vi "toStringArray.vi"(8 "error in (no error)":errorcluster, 11 "ScriptEvent in":refnum<class "ScriptEvent.lvclass">) -> (0 "error out":errorcluster, 2 "eventStringArray":string[](array[string]), 3 "ScriptEvent out":refnum<class "ScriptEvent.lvclass">)   [LabVIEW 2011, in "Tools.lvlib" / "Scripting.lvlib" / "ScriptEvent.lvclass"]
uses:
  ScriptEvent.lvclass
  ScriptEvent.lvclass/ScriptEvent.ctl
  DatabaseHelpers/Database Objects/Channel/Channel.lvclass
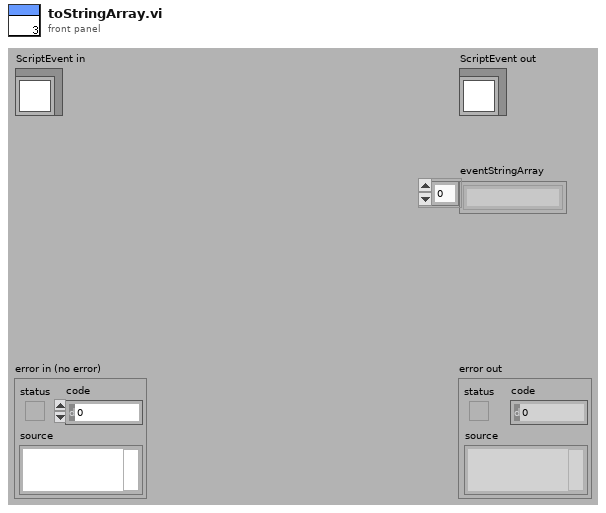
[diagram p1: front panel]
types:
  T1 = enum16{"changeValue", "pulse", "clock", "rampUp", "rampDown", "singleTone", "singleToneRamp", "playFile", "rf", "rfRamp", "delay"}
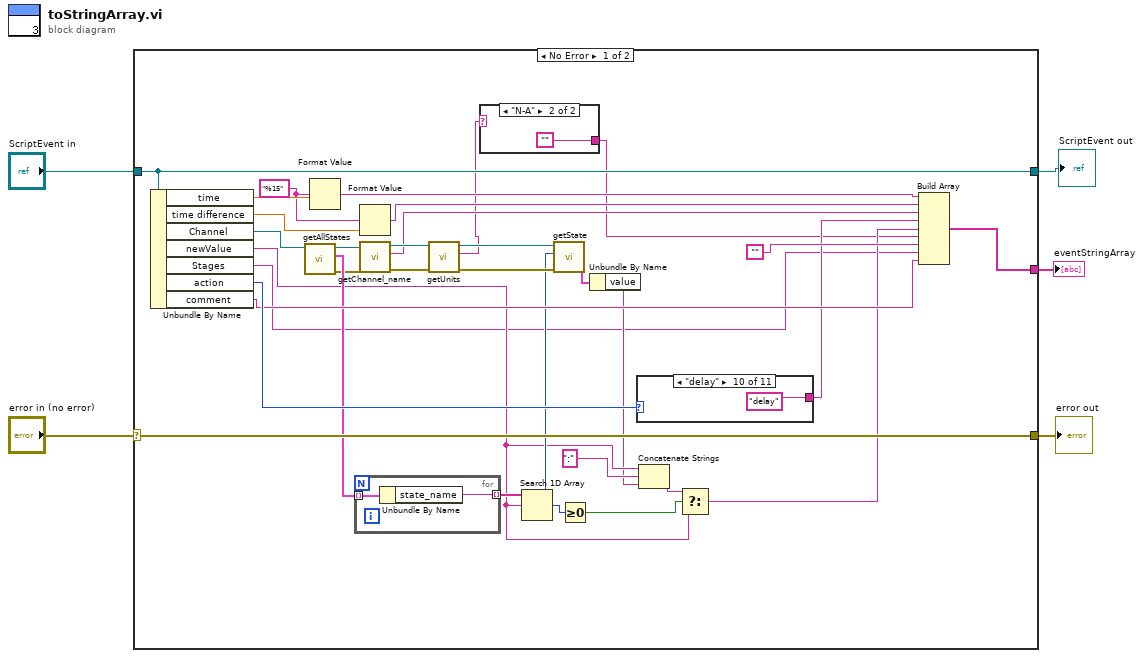
[diagram p0: block diagram]
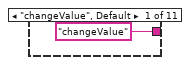
[diagram p3: hidden frame]
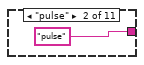
[diagram p4: hidden frame]
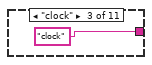
[diagram p5: hidden frame]
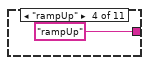
[diagram p6: hidden frame]
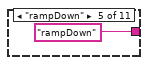
[diagram p7: hidden frame]
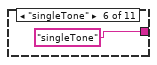
[diagram p8: hidden frame]
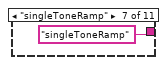
[diagram p9: hidden frame]
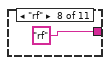
[diagram p10: hidden frame]
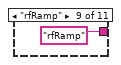
[diagram p11: hidden frame]
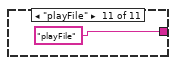
[diagram p12: hidden frame]
diagram:
  n1 = case shown="No Error" "error in (no error)" {
    selector: "error in (no error)" -> [w38 w55]
    tunnel: [w38 w55] -> w4
    tunnel: [w37 w54] -> w2
    tunnel: "ScriptEvent in" -> [w37 w54]
    tunnel: [w26 _] -> w1
    frame No Error {
      w34 = "%15"
      n2 = Unbundle By Name(w37) -> ("time"=w36:dbl, "time difference"=w35:dbl, "Channel"=w21:refnum<class "Channel.lvclass">, "newValue"=w10:string, "Stages"=w6:string, "action"=w28:T1, "comment"=w27:string)
      n3 = call "getAllStates.vi"("Channel.lvclass in"=w21) -> ("error out"=w20:errorcluster, "states"=w23:cluster{"state_name":string, "value":string}[], "Channel.lvclass out"=w22:refnum<class "Channel.lvclass">)  [unwired: 8 in]
      n4 = Format Value(format string=w34, value (0)=w36) -> (output string=w31:string)  [unwired: 1 in]
      n5 = for {
        tunnel: w23 -> [w42] mode=indexing
        tunnel: [w41] -> w19 mode=indexing
        n6 = Unbundle By Name(w42) -> ("state_name"=w41:string)
      }
      n7 = Format Value(format string=w34, value (0)=w35) -> (output string=w30:string)  [unwired: 1 in]
      n8 = call "getChannel_name.vi"("error in (no error)"=w20, "Channel.lvclass in"=w22) -> ("error out"=w32:errorcluster, "channel_name"=w29:string, "Channel.lvclass out"=w33:refnum<class "Channel.lvclass">)  [unwired: 7 in]
      n9 = call-dynamic "getUnits.vi"("error in (no error)"=w32, "Channel.lvclass in"=w33) -> ("error out"=w13:errorcluster, "units"=w8:string, "Channel.lvclass out"=w14:refnum<class "Channel.lvclass">)  [unwired: 7 in]
      n10 = case shown="\"N-A\"" w8 {
        selector: w8 -> [w39 _]
        tunnel: [w39 ""] -> w7
        frame Default {
        }
        frame "N-A" {
        }
      }
      n11 = Search 1D Array(1D array=w19, element=w10) -> (index of element=w12:i32)  [unwired: 1 in]
      n12 = call "getState.vi"("error in (no error)"=w13, "index"=w12, "Channel.lvclass in"=w14) -> ("state"=w11:cluster{"state_name":string, "value":string})  [unwired: 6 in, 2 out]
      n13 = Greater Or Equal To 0?(x=w12) -> (x >= 0?=w16:bool)
      n14 = Unbundle By Name(w11) -> ("value"=w9:string)
      n15 = case shown="\"delay\"" w28 {
        tunnel: ["changeValue" "pulse" "clock" "rampUp" "rampDown" "singleTone" "singleToneRamp" "rf" "rfRamp" "delay" "playFile"] -> w24
        frame "changeValue", Default {
        }
        frame "pulse" {
        }
        frame "clock" {
        }
        frame "rampUp" {
        }
        frame "rampDown" {
        }
        frame "singleTone" {
        }
        frame "singleToneRamp" {
        }
        frame "rf" {
        }
        frame "rfRamp" {
        }
        frame "delay" {
        }
        frame "playFile" {
        }
      }
      n16 = Concatenate Strings(w10, ":", w9) -> (w17:string)
      n17 = Select(t=w17, s=w16, f=w10) -> (s? t:f=w15:string)
      n18 = Build Array(w31, w30, w29, w24, w15, w7, "", w6, w27) -> (w26:string[])
    }
    frame Error {
    }
  }
  "error out" <- w4
  "ScriptEvent out" <- w2
  "eventStringArray" <- w1
